vi "FPGA Sampling Rate Ratio.vi"(7 "nominal Fs (50000 Hz)":u32=50000, 9 "timestamp valid? (T)":bool=TRUE, 11 "timestamp [s]":fxp<+,64,32>) -> (3 "nominal Fs/actual Fs":fxp<+,64,32> format="%#_19g")   [LabVIEW 2014, in "NI_EP_PMU_FPGA.lvlib"]
doc: "Calculates the ratio of the nominal sample rate to the actual sample rate of the data acquisition module as the correction parameters for frequency calculation."
uses:
  <vilib>/addons/Electrical Power/PMU/NI_EP_PMU_FPGA.lvlib
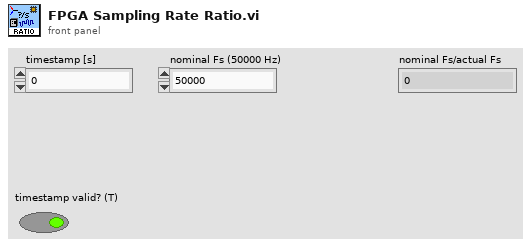
[diagram p1: front panel]
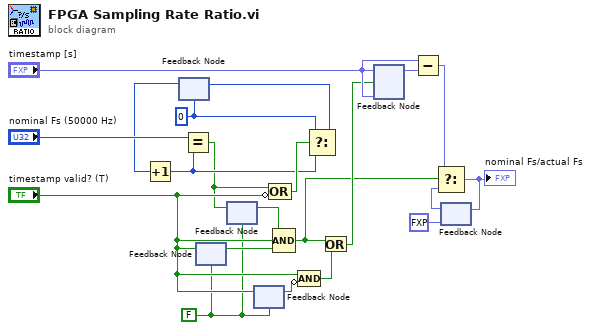
[diagram p0: block diagram]
diagram:
  w4 = FALSE ("timestamp valid? (T)")
  w21 = u32 0 ("s")
  n1 = feedback #1(w21) -> (w9:u32)
  n2 = Increment(x=w9) -> (x+1=w8:u32)
  n3 = Equal?(x="nominal Fs (50000 Hz)", y=w8) -> (x = y?=w5:bool)
  n4 = feedback #2(w4) -> (w7:bool)
  n5 = feedback-in #2("timestamp valid? (T)") -> ()
  n6 = feedback #3(w4) -> (w3:bool)
  n7 = feedback-in #3(w5) -> ()
  n8 = feedback #4(w4) -> (w12:bool)
  n9 = feedback-in #4("timestamp valid? (T)") -> ()
  n10 = Compound Arithmetic op=OR(w5, invert "timestamp valid? (T)") -> (w10:bool)
  n11 = Compound Arithmetic op=AND(w3, "timestamp valid? (T)", w7) -> (w1:bool)
  n12 = Compound Arithmetic op=AND("timestamp valid? (T)", invert w12) -> (w11:bool)
  n13 = Select(t=w21, s=w10, f=w8) -> (s? t:f=w20:u32)
  n14 = feedback-in #1(w20) -> ()
  n15 = Or(x=w1, y=w11) -> (x .or. y?=w2:bool)
  n16 = feedback #5("timestamp [s]") -> (w18:fxp<+,64,32>)
  n17 = feedback-in #5("timestamp [s]", w2) -> ()
  n18 = Subtract(x="timestamp [s]", y=w18) -> (x-y=w16:fxp<+,64,32>)
  n19 = feedback #6(fxp<+,64,32> 1.0) -> (w15:fxp<+,64,32>)
  n20 = Select(t=w16, s=w1, f=w15) -> (s? t:f=w13:fxp<+,64,32>)
  "nominal Fs/actual Fs" <- w13
  n21 = feedback-in #6(w13) -> ()
